vi "int to enum.vi"() -> ()   [LabVIEW 2016]
panel:
  out "Input":i32
  out "Output":T1(ring)
  out "Enum":T1(ring)
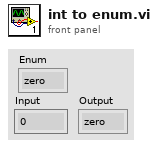
[diagram p1: front panel]
types:
  T1 = enum16{"zero", "one", "two", "three", "four", "five"}
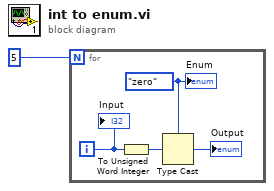
[diagram p0: block diagram]
diagram:
  n1 = for {
    N: 5 ("Numeric") -> [_]
    i -> [w3]
    w5 = T1."zero"
    n2 = To Unsigned Word Integer(number=w3) -> (unsigned 16bit integer=w2:u16)
    n3 = Type Cast(type=w5, x=w2) -> (*(type *) &x=→"Output":T1)
    "Enum" <- w5
    "Input" <- w3
  }
